vi "1-1.vi"() -> ()   [LabVIEW 2019, in "1.lvlib"]
uses:
  <vilib>/Utility/file.llb/Read Delimited Spreadsheet (I64).vi
  1.lvlib
panel:
  out "index":i32
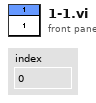
[diagram p1: front panel]
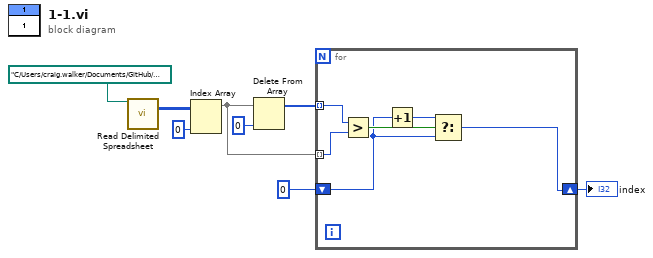
[diagram p0: block diagram]
diagram:
  n1 = call-poly <vilib>:"Read Delimited Spreadsheet.vi"("file path (dialog if empty)"=path "C:/Users/craig.walker/Documents/GitHub/lv2019-Advent-of-Code-2021/1/input.txt") -> ("all rows"=w6:i64[][])  [unwired: 9 in, 5 out]
  n2 = Index Array(array=w6, index (col)=0 ("disabled index (col)")) -> (element=w4:i64[])  [unwired: 1 in]
  n3 = Delete From Array(array=w4, index=0) -> (array with subset deleted=w3:i64[])  [unwired: 1 in, 1 out]
  n4 = for {
    tunnel: w4 -> [w13] mode=indexing
    tunnel: w3 -> [w14] mode=indexing
    shift-right: [w11] -> w1
    shift-left: 0 ("index") -> [w10]
    n5 = Greater?(x=w14, y=w13) -> (0:w12:bool)
    n6 = Increment(x=w10) -> (x+1=w9:i32)
    n7 = Select(t=w9, s=w12, f=w10) -> (s? t:f=w11:i32)
  }
  "index" <- w1
